vi "KM101_Change_nm_step.vi"(3 "DataIn":dbl, 4 "方式":enum16{"Step-nm", "nm-Step"}(ring), 5 "电机":T1) -> (0 "DataOut":dbl)   [LabVIEW 2018]
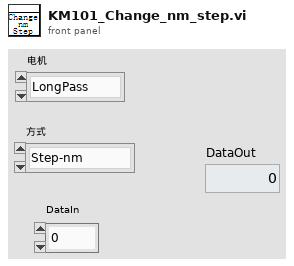
[diagram p1: front panel]
types:
  T1 = typedef "电机枚举.ctl" = enum16{"LongPass", "ShortPass"}
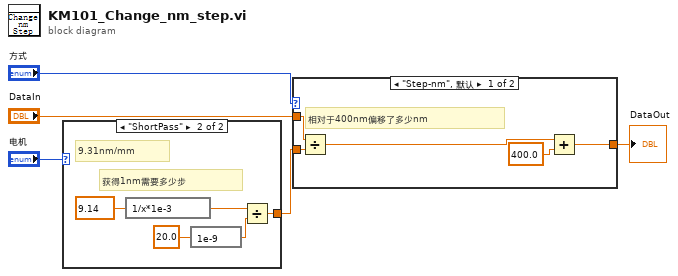
[diagram p0: block diagram]
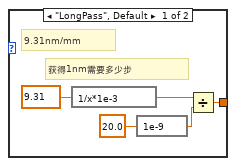
[diagram p2: hidden frame]
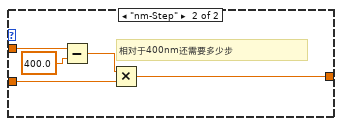
[diagram p3: hidden frame]
diagram:
  n1 = case shown="\"ShortPass\"" "电机" {
    tunnel: [w6 w11] -> w1
    frame "LongPass", Default {
      # "获得1nm需要多少步"
      # "9.31nm/mm"
      n2 = expression code="1/x*1e-3"(9.31) -> (w10:dbl)
      n3 = expression code="1e-9"(20.0) -> (w7:dbl)
      n4 = Divide(x=w10, y=w7) -> (x/y=w6:dbl)
    }
    frame "ShortPass" {
      # "获得1nm需要多少步"
      # "9.31nm/mm"
      n5 = expression code="1/x*1e-3"(9.14) -> (w15:dbl)
      n6 = expression code="1e-9"(20.0) -> (w12:dbl)
      n7 = Divide(x=w15, y=w12) -> (x/y=w11:dbl)
    }
  }
  n8 = case shown="\"Step-nm\", 默认" "方式" {
    tunnel: "DataIn" -> [w20 w25]
    tunnel: [w16 w23] -> w3
    tunnel: w1 -> [w19 w24]
    frame "Step-nm", Default {
      # "相对于400nm偏移了多少nm"
      n9 = Divide(x=w20, y=w19) -> (x/y=w18:dbl)
      n10 = Add(x=w18, y=400.0) -> (x+y=w16:dbl)
    }
    frame "nm-Step" {
      # "相对于400nm还需要多少步"
      n11 = Subtract(x=w25, y=400.0) -> (x-y=w22:dbl)
      n12 = Multiply(x=w22, y=w24) -> (x*y=w23:dbl)
    }
  }
  "DataOut" <- w3
